vi "Detect Collision with HAB.vi"(1 "Right Current":dbl, 2 "Right Velocity":dbl, 3 "Left Current":dbl, 4 "Left Velocity":dbl) -> (0 "HIT WALL":bool)   [LabVIEW 2018]
panel:
  in  "Current Threshold":dbl=8.0
  in  "Velocity Threshold":dbl=20.0
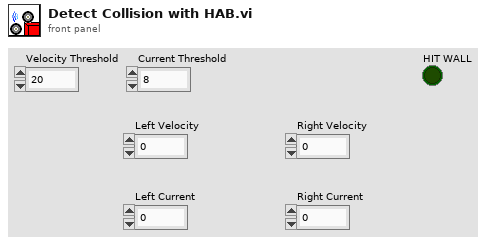
[diagram p1: front panel]
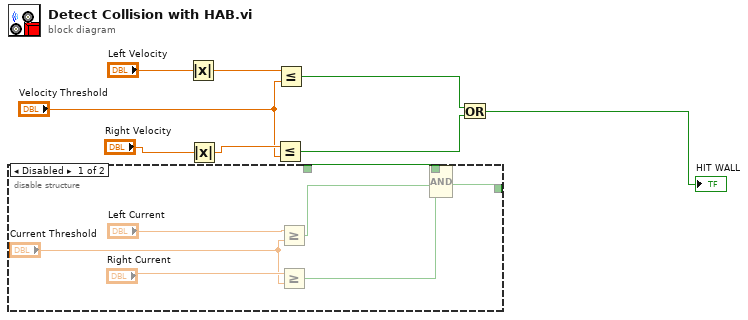
[diagram p0: block diagram]
diagram:
  n1 = disable-structure shown="Disabled" {
    disable-tunnel: _ -> [w14 _]
    disable-tunnel: _ -> [w13 _]
    disable-tunnel: [w10 _] -> _
    frame Disabled {
      n2 = Greater Or Equal?(x="Left Current", y="Current Threshold") -> (x >= y?=w12:bool)
      n3 = Greater Or Equal?(x="Right Current", y="Current Threshold") -> (x >= y?=w11:bool)
      n4 = Compound Arithmetic op=AND(w14, w13, w12, w11) -> (w10:bool)
    }
    frame Enabled {
    }
  }
  n5 = Absolute Value(x="Left Velocity") -> (abs(x)=w5:dbl)
  n6 = Absolute Value(x="Right Velocity") -> (abs(x)=w7:dbl)
  n7 = Less Or Equal?(x=w7, y="Velocity Threshold") -> (x <= y?=w2:bool)
  n8 = Less Or Equal?(x=w5, y="Velocity Threshold") -> (x <= y?=w3:bool)
  n9 = Or(x=w3, y=w2) -> (x .or. y?=→"HIT WALL":bool)
